vi "Write Step State.vi"(8 "error in (no error)":errorcluster, 10 "Step State":T1, 11 "Step in":refnum<class "Step.lvclass">) -> (0 "error out":errorcluster, 3 "Step out":refnum<class "Step.lvclass">)   [LabVIEW 2015, in "Step.lvclass"]
uses:
  Step.lvclass
  StepState.ctl
  Step Status.ctl
  Step Flow Control.ctl
  Step.lvclass/Step.ctl
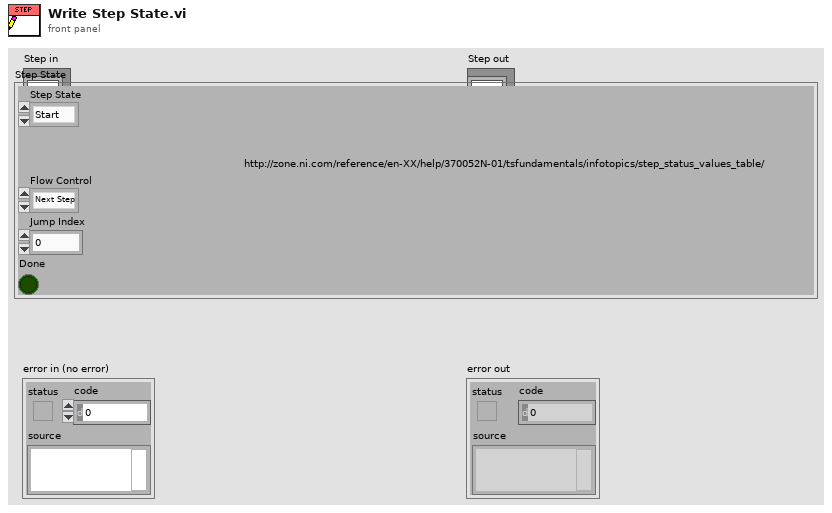
[diagram p1: front panel]
types:
  T1 = typedef "Step.lvclass/StepState.ctl" = cluster{"Step State":T2, "Flow Control":T3, "Jump Index":i32, "Done":bool}
  T2 = typedef "Step.lvclass/Step Status.ctl" = enum16{"Start", "Passed", "Failed", "Error", "Done", "Terminated", "Skipped", "Running"}
  T3 = typedef "Step.lvclass/Step Flow Control.ctl" = enum16{"Next Step", "Jump"}
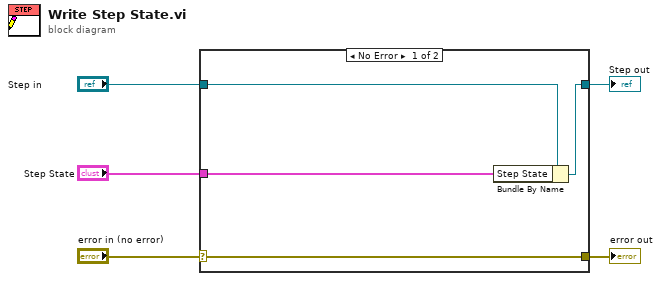
[diagram p0: block diagram]
diagram:
  n1 = case shown="No Error" "error in (no error)" {
    selector: "error in (no error)" -> [w9 w10]
    tunnel: [w9 w10] -> w4
    tunnel: [w7 w11] -> w2
    tunnel: "Step in" -> [w8 w11]
    tunnel: "Step State" -> [w6 _]
    frame No Error {
      n2 = Bundle By Name(cluster=w8, "Step State"=w6) -> (w7:refnum<class "Step.lvclass">)
    }
    frame Error {
    }
  }
  "error out" <- w4
  "Step out" <- w2
